vi "Parse List.vi"(11 "String":string) -> (3 "List":T1[](array[typedef]))   [LabVIEW 2020]
uses:
  Control 2.ctl
  ENUM_Item Type.ctl
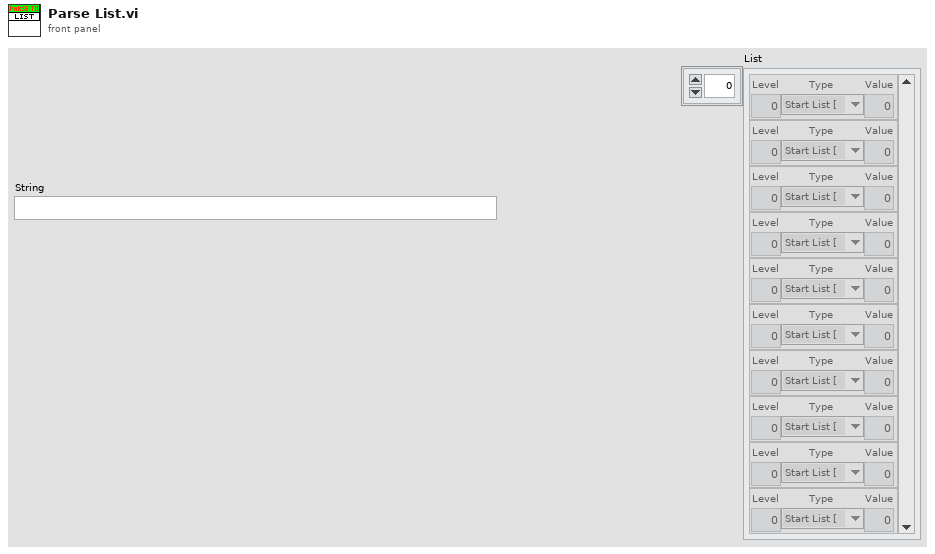
[diagram p1: front panel]
types:
  T1 = typedef "Control 2.ctl" = cluster{"Level":i32, "Type":T2, "Value":i32}
  T2 = typedef "ENUM_Item Type.ctl" = enum16{"Start List [", "Integer", "End List ]"}
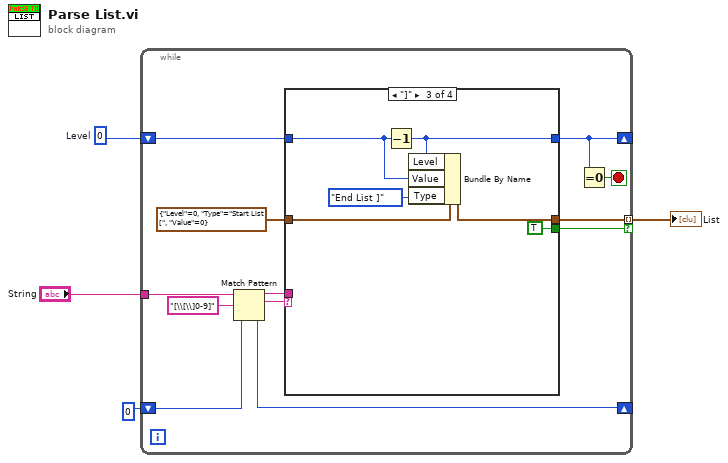
[diagram p0: block diagram]
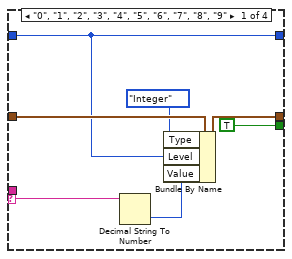
[diagram p2: hidden frame]
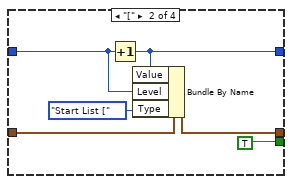
[diagram p3: hidden frame]
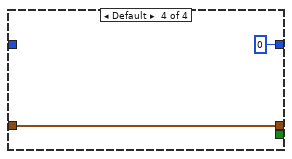
[diagram p4: hidden frame]
diagram:
  w3 = 0  # Level
  n1 = while {
    shift-right: [w11] -> _
    shift-left: w3 -> [w12]
    shift-right: [w14] -> _
    shift-left: 0 ("offset (0)") -> [w5]
    tunnel: [w8] -> w1 mode=indexing if=w7
    tunnel: "String" -> [w15]
    stop <- w16 stop-if-true
    n2 = Match Pattern(string=w15, regular expression="[\\[\\]0-9]", offset (0)=w5) -> (before substring=w6:string, match substring=w10:string, offset past match=w14:i32)  [unwired: 1 out]
    n3 = case shown="\"]\"" w10 {
      selector: w10 -> [w17 _ _ _]
      tunnel: w12 -> [w20 w27 w33 _]
      tunnel: [w20 w25 w31 0 ("Level")] -> w11
      tunnel: T1 {"Level"=0, "Type"=enum."Start List [", "Value"=0} ("Character") -> [w22 w28 w34 w36]
      tunnel: [w21 w29 w35 w36] -> w8
      tunnel: [TRUE TRUE TRUE _] -> w7
      tunnel: w6 -> [_ _ _ _]
      frame "0", "1", "2", "3", "4", "5", "6", "7", "8", "9" {
        n4 = Decimal String To Number(string=w17) -> (number=w18:i32)  [unwired: 2 in, 1 out]
        n5 = Bundle By Name(cluster=w22, "Type"=ENUM_Item_Type."Integer", "Level"=w20, "Value"=w18) -> (w21:T1)
      }
      frame "[" {
        n6 = Increment(x=w27) -> (x+1=w25:i32)
        n7 = Bundle By Name(cluster=w28, "Value"=w25, "Level"=w27, "Type"=ENUM_Item_Type."Start List [") -> (w29:T1)
      }
      frame "]" {
        n8 = Decrement(x=w33) -> (x-1=w31:i32)
        n9 = Bundle By Name(cluster=w34, "Level"=w31, "Value"=w33, "Type"=ENUM_Item_Type."End List ]") -> (w35:T1)
      }
      frame Default {
      }
    }
    n10 = Equal To 0?(x=w11) -> (x = 0?=w16:bool)
  }
  "List" <- w1
